vi "Get FPGA Reference.vi"(8 "error in (no error)":errorcluster, 11 "LIA Host Interface in":refnum<class "LIA Host Interface.lvclass">) -> (0 "error out":errorcluster, 2 "Properties:FPGA Session":refnum<k20>, 3 "LIA Host Interface out":refnum<class "LIA Host Interface.lvclass">)   [LabVIEW 2017, in "LIA Debugging.lvclass"]
uses:
  LIA Debugging.lvclass
  Program Files (x86)/National Instruments/LabVIEW 2017/examples/Lock-In Amplifier/lib/interface/Interface/LIA Host Interface.lvclass
  Program Files (x86)/National Instruments/LabVIEW 2017/examples/Lock-In Amplifier/lib/interface/Interface FPGA/LIA Host Interface FPGA.lvclass
  Program Files (x86)/National Instruments/LabVIEW 2017/examples/Lock-In Amplifier/lib/interface/Interface FPGA/Properties/FpgaSession_GET.vi
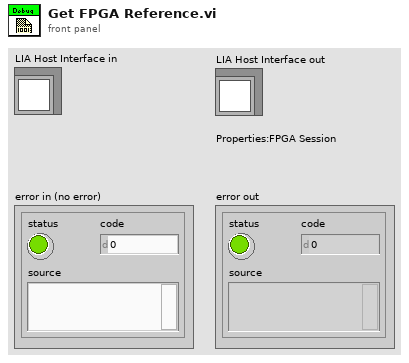
[diagram p1: front panel]
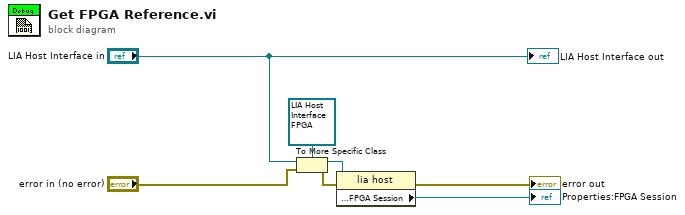
[diagram p0: block diagram]
diagram:
  n1 = To More Specific Class(target class=refnum<class "LIA Host Interface FPGA.lvclass"> refnum ("lia host"), reference="LIA Host Interface in", error in="error in (no error)") -> (specific class reference=w2:refnum<class "LIA Host Interface FPGA.lvclass">, error out=w6:errorcluster)
  n2 = property class="lia host"(reference=w2, error in=w6) -> (error out=→"error out":errorcluster, "Properties:FPGA Session"=→"Properties:FPGA Session":refnum<k20>)  [unwired: 1 out]
  "LIA Host Interface out" <- "LIA Host Interface in"
